vi "edit_coating(in).vi"(0 "Path":string) -> ()   [LabVIEW 2009]
uses:
  <vilib>/Utility/file.llb/Read From Spreadsheet File (string).vi
panel:
  in  "Recipe List":i32(listbox)
  out "error out":errorcluster
  out "Path Array":string[](array[string])
  out "Recipe":string[](array[string])
  in  "Coating Name :":string
  in  "Add Recipe":bool
  in  "ok":bool
  in  "cancel":bool
  in  "delete":bool
  in  "Move up":bool
  in  "Move down":bool
  in  "Coating":i32(listbox)
  out "OKTO":bool
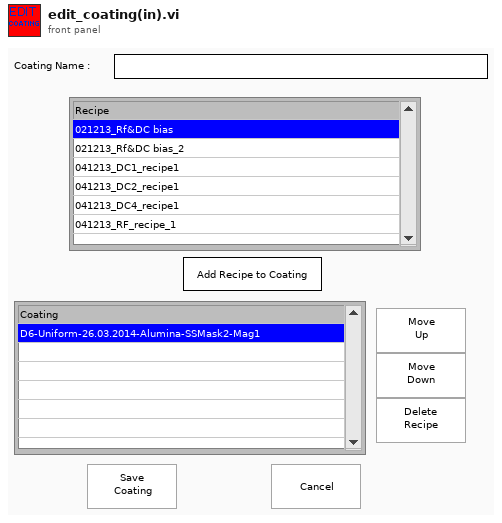
[diagram p1: front panel]
types:
  T1 = enum16{"open", "replace", "create", "open or create", "replace or create", "replace or create with confirmation"}
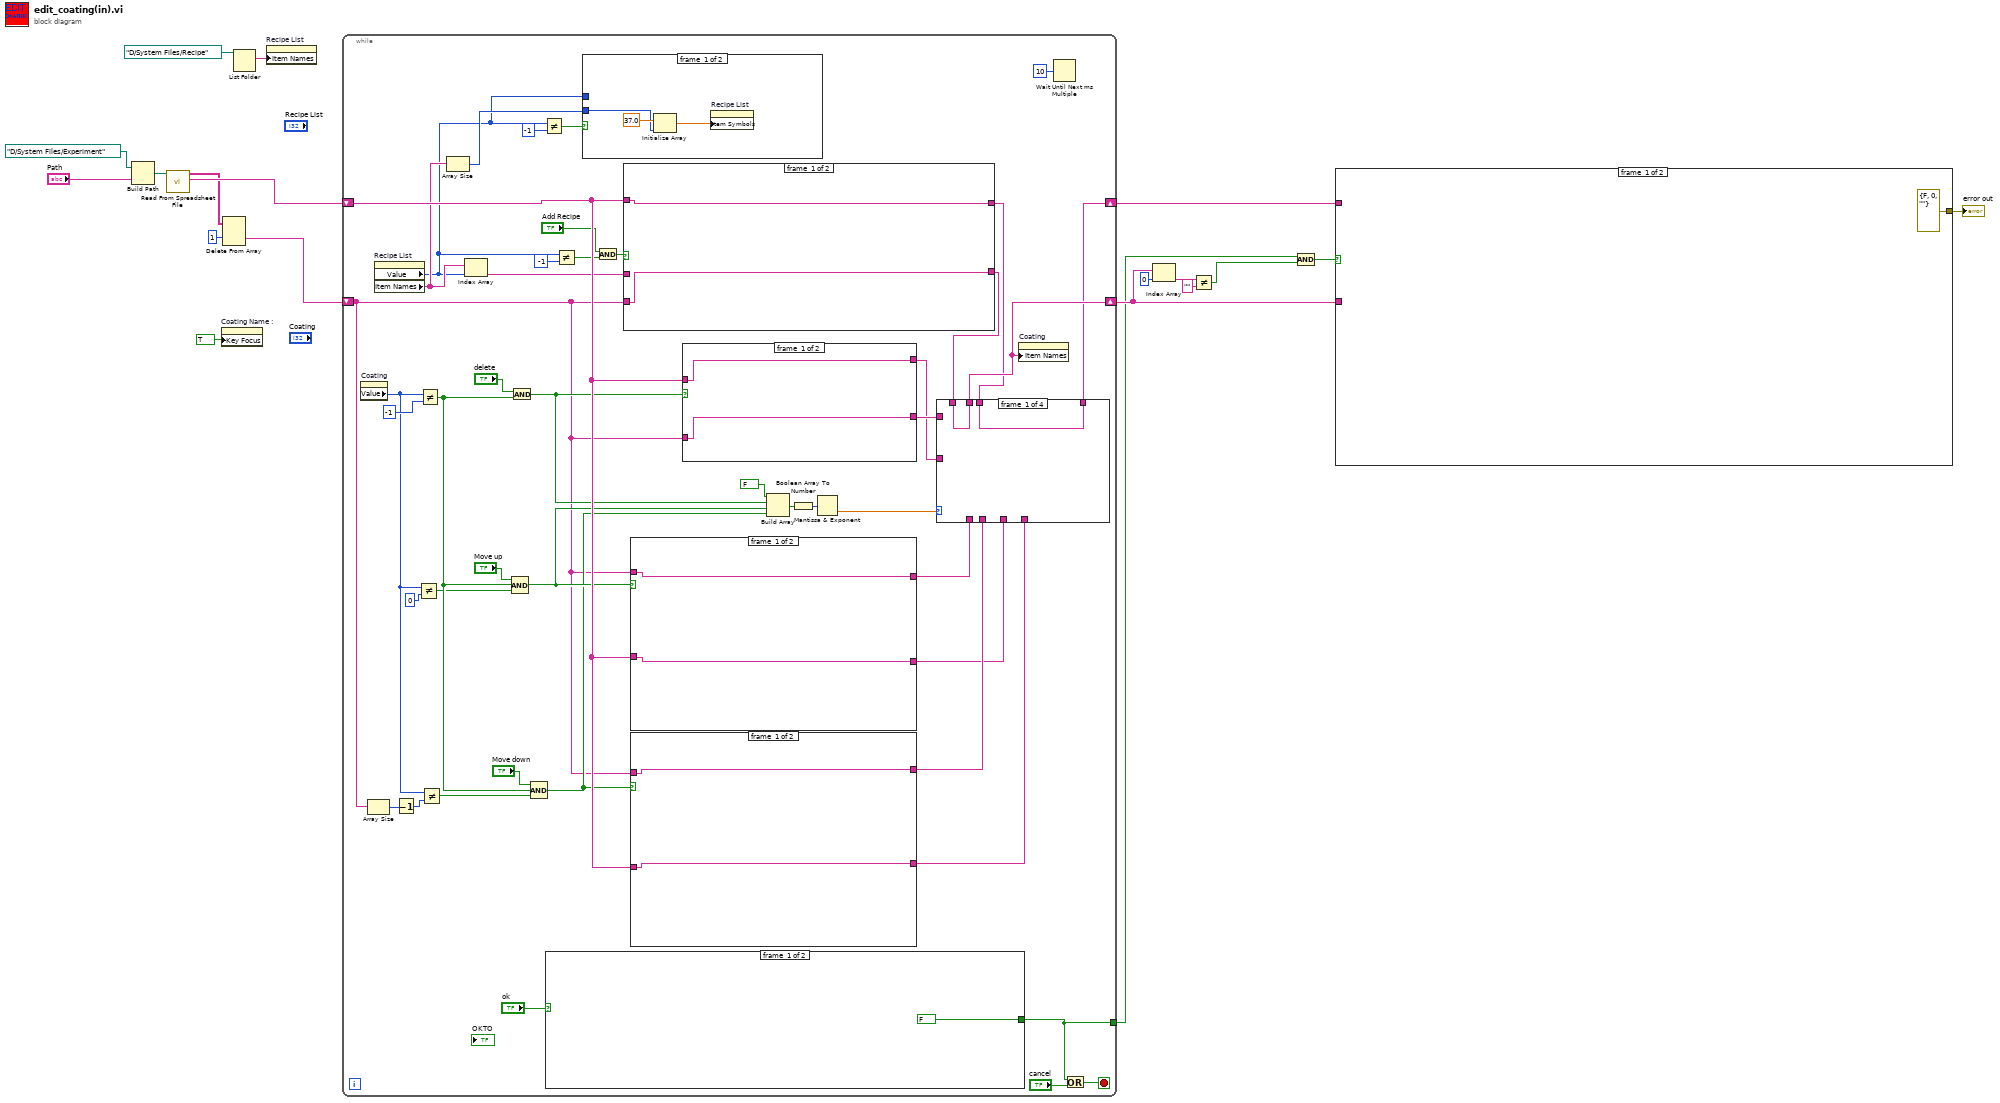
[diagram p0: block diagram]
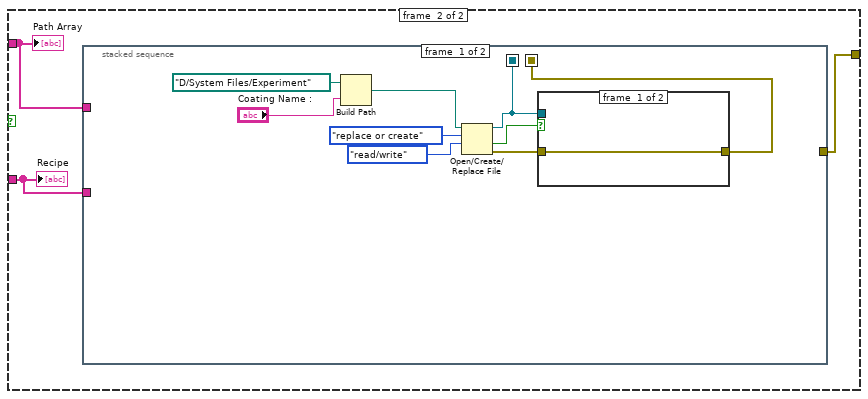
[diagram p2: hidden frame]
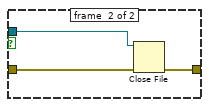
[diagram p3: hidden frame]
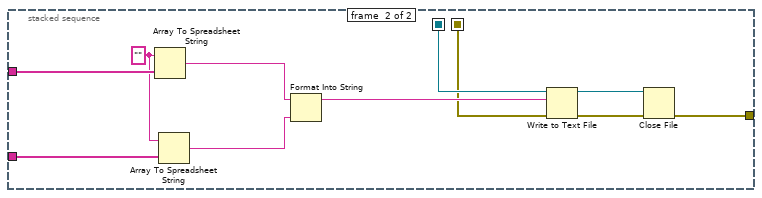
[diagram p4: hidden frame]
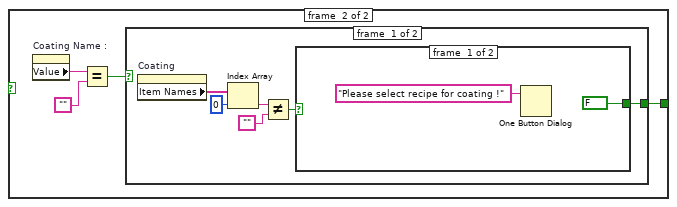
[diagram p5: hidden frame]
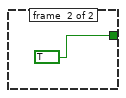
[diagram p6: hidden frame]
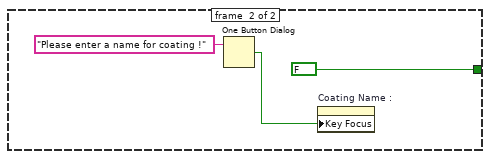
[diagram p7: hidden frame]
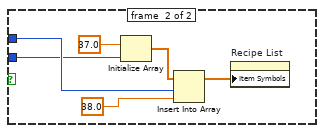
[diagram p8: hidden frame]
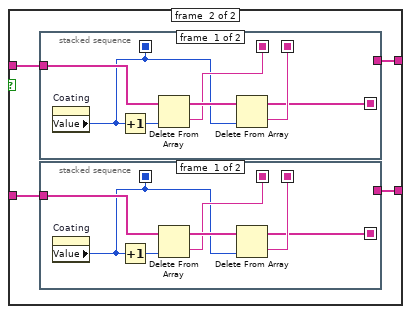
[diagram p12: hidden frame]
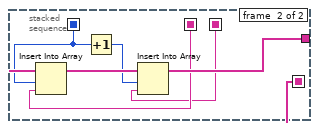
[diagram p13: hidden frame]
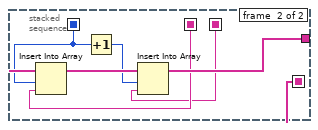
[diagram p14: hidden frame]
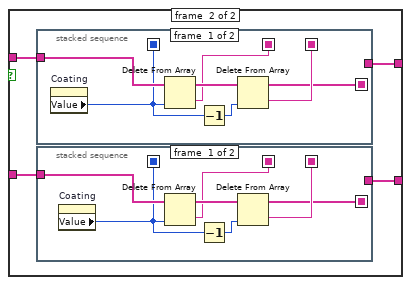
[diagram p15: hidden frame]
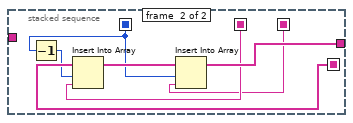
[diagram p16: hidden frame]
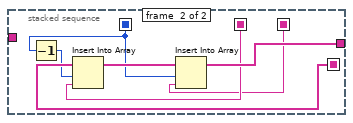
[diagram p17: hidden frame]
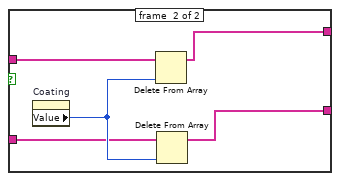
[diagram p18: hidden frame]
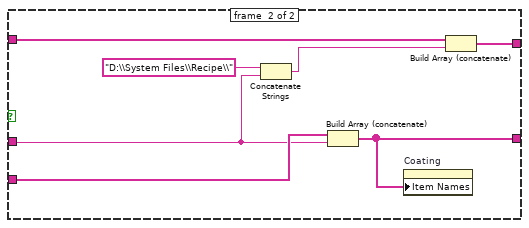
[diagram p19: hidden frame]
diagram:
  n1 = Build Path(base path=path "D:/System Files/Experiment", name or relative path="Path") -> (appended path=w19:path)
  n2 = call-poly <vilib>:"Read From Spreadsheet File.vi"("file path (dialog if empty)"=w19) -> ("first row"=w4:string[], "all rows"=w2:string[][])  [unwired: 6 in, 3 out]
  n3 = property on="Coating Name :" class="Str"("Key Focus"=TRUE) -> ()  [unwired: 2 in, 2 out]
  n4 = Delete From Array(array=w2, index (row)=1) -> (deleted portion=w1:string[])  [unwired: 2 in, 1 out]
  n5 = List Folder(path=path "D:/System Files/Recipe") -> (filenames=w8:string[])  [unwired: 3 in, 3 out]
  n6 = property on="Recipe List" class="LstBox (strict)"("Item Names"=w8) -> ()  [unwired: 2 in, 2 out]
  n7 = while {
    shift-right: [w51] -> w16
    shift-left: w4 -> [w54]
    shift-right: [w55] -> w15
    shift-left: w1 -> [w35]
    tunnel: [w21] -> w5
    stop <- w63 stop-if-true
    n8 = property on="Coating" class="LstBox (strict)"() -> ("Value"=w36:i32)  [unwired: 2 in, 2 out]
    n9 = Array Size(array=w35) -> (size(s)=w34:i32)
    n10 = property on="Recipe List" class="LstBox (strict)"() -> ("Value"=w23:i32, "Item Names"=w30:string[])  [unwired: 2 in, 2 out]
    n11 = Decrement(x=w34) -> (x-1=w33:i32)
    n12 = Not Equal?(x=w36, y=0) -> (x != y?=w38:bool)
    n13 = Not Equal?(x=w36, y=-1) -> (x != y?=w42:bool)
    n14 = Not Equal?(x=w36, y=w33) -> (x != y?=w37:bool)
    n15 = Array Size(array=w30) -> (size(s)=w28:i32)
    n16 = Index Array(array=w30, index=w23) -> (element=w32:string)
    n17 = And(x="delete", y=w42) -> (x .and. y?=w45:bool)
    n18 = Compound Arithmetic op=AND("Move up", w42, w38) -> (w43:bool)
    n19 = Compound Arithmetic op=AND("Move down", w42, w37) -> (w40:bool)
    n20 = Not Equal?(x=w23, y=-1) -> (x != y?=w29:bool)
    n21 = case shown="True" "ok" {
      tunnel: [FALSE w66] -> w21
      frame #0 {
      }
      frame #1 {
        n22 = property on="Coating Name :" class="Str"() -> ("Value"=w68:string)  [unwired: 2 in, 2 out]
        n23 = Equal?(x=w68, y="") -> (x = y?=w67:bool)
        n24 = case shown="True" w67 {
          tunnel: [w70 FALSE] -> w66
          frame #0 {
            n25 = property on="Coating" class="LstBox (strict)"() -> ("Item Names"=w73:string[])  [unwired: 2 in, 2 out]
            n26 = Index Array(array=w73, index=0) -> (element=w75:string)
            n27 = Not Equal?(x=w75, y="") -> (x != y?=w71:bool)
            n28 = case shown="False" w71 {
              tunnel: [FALSE TRUE] -> w70
              frame #0 {
                n29 = One Button Dialog(message="Please select recipe for coating !") -> ()  [unwired: 1 in, 1 out]
              }
              frame #1 {
              }
            }
          }
          frame #1 {
            n30 = One Button Dialog(message="Please enter a name for coating !") -> (true=w79:bool)  [unwired: 1 in]
            n31 = property on="Coating Name :" class="Str"("Key Focus"=w79) -> ()  [unwired: 2 in, 2 out]
          }
        }
      }
    }
    n32 = Not Equal?(x=w23, y=-1) -> (x != y?=w24:bool)
    n33 = case shown="False" w29 {
      tunnel: w23 -> [_ w87]
      tunnel: w28 -> [w83 w86]
      frame #0 {
        n34 = Initialize Array(37.0 ("element"), w83) -> (w82:dbl[])
        n35 = property on="Recipe List" class="LstBox (strict)"("Item Symbols"=w82) -> ()  [unwired: 2 in, 2 out]
      }
      frame #1 {
        n36 = Initialize Array(37.0 ("element"), w86) -> (w90:dbl[])
        n37 = Insert Into Array(array=w90, index=w87, new element=38.0 ("element")) -> (w85:dbl[])
        n38 = property on="Recipe List" class="LstBox (strict)"("Item Symbols"=w85) -> ()  [unwired: 2 in, 2 out]
      }
    }
    n39 = And(x="Add Recipe", y=w24) -> (x .and. y?=w26:bool)
    n40 = case shown="True" w26 {
      tunnel: [w175 w180] -> w52
      tunnel: [w174 w179] -> w53
      tunnel: w35 -> [w174 w182]
      tunnel: w54 -> [w175 w181]
      tunnel: w32 -> [_ w177]
      frame #0 {
      }
      frame #1 {
        n41 = Concatenate Strings("D:\\System Files\\Recipe\\" ("string"), w177) -> (w176:string)
        n42 = Build Array (concatenate)(w182, w177) -> (w179:string[])
        n43 = property on="Coating" class="LstBox (strict)"("Item Names"=w179) -> ()  [unwired: 2 in, 2 out]
        n44 = Build Array (concatenate)(w181, w176) -> (w180:string[])
      }
    }
    n45 = case shown="True" w43 {
      tunnel: w35 -> [w134 w138]
      tunnel: [w134 w137] -> w57
      tunnel: w54 -> [w133 w136]
      tunnel: [w133 w135] -> w50
      frame #0 {
      }
      frame #1 {
        n46 = stacked-sequence {
          seq-local: [w156 _] -> [_ w161]
          seq-local: [w155 _] -> [_ w160]
          seq-local: [w154 _] -> [_ w166]
          seq-local: [w153 _] -> [_ w163]
          tunnel: w138 -> [w159 _]
          tunnel: [_ w164] -> w137
          frame #0 {
            n47 = property on="Coating" class="LstBox (strict)"() -> ("Value"=w153:i32)  [unwired: 2 in, 2 out]
            n48 = Delete From Array(array=w159, index=w153) -> (deleted portion=w156:string, array with subset deleted=w158:string[])  [unwired: 1 in]
            n49 = Decrement(x=w153) -> (x-1=w157:i32)
            n50 = Delete From Array(array=w158, index=w157) -> (deleted portion=w155:string, array with subset deleted=w154:string[])  [unwired: 1 in]
          }
          frame #1 {
            n51 = Decrement(x=w163) -> (x-1=w162:i32)
            n52 = Insert Into Array(array=w166, index=w162, new element=w161) -> (w165:string[])
            n53 = Insert Into Array(array=w165, index=w163, new element=w160) -> (w164:string[])
          }
        }
        n54 = stacked-sequence {
          seq-local: [w142 _] -> [_ w147]
          seq-local: [w141 _] -> [_ w146]
          seq-local: [w140 _] -> [_ w152]
          seq-local: [w139 _] -> [_ w149]
          tunnel: w136 -> [w145 _]
          tunnel: [_ w150] -> w135
          frame #0 {
            n55 = property on="Coating" class="LstBox (strict)"() -> ("Value"=w139:i32)  [unwired: 2 in, 2 out]
            n56 = Delete From Array(array=w145, index=w139) -> (deleted portion=w142:string, array with subset deleted=w144:string[])  [unwired: 1 in]
            n57 = Decrement(x=w139) -> (x-1=w143:i32)
            n58 = Delete From Array(array=w144, index=w143) -> (deleted portion=w141:string, array with subset deleted=w140:string[])  [unwired: 1 in]
          }
          frame #1 {
            n59 = Decrement(x=w149) -> (x-1=w148:i32)
            n60 = Insert Into Array(array=w152, index=w148, new element=w147) -> (w151:string[])
            n61 = Insert Into Array(array=w151, index=w149, new element=w146) -> (w150:string[])
          }
        }
      }
    }
    n62 = case shown="True" w40 {
      tunnel: w35 -> [w100 w104]
      tunnel: [w100 w103] -> w56
      tunnel: w54 -> [w99 w102]
      tunnel: [w99 w101] -> w48
      frame #0 {
      }
      frame #1 {
        n63 = stacked-sequence {
          seq-local: [w121 _] -> [_ w129]
          seq-local: [w123 _] -> [_ w128]
          seq-local: [w122 _] -> [_ w132]
          seq-local: [w119 _] -> [_ w126]
          tunnel: w104 -> [w124 _]
          tunnel: [_ w131] -> w103
          frame #0 {
            n64 = property on="Coating" class="LstBox (strict)"() -> ("Value"=w119:i32)  [unwired: 2 in, 2 out]
            n65 = Increment(x=w119) -> (x+1=w120:i32)
            n66 = Delete From Array(array=w124, index=w120) -> (deleted portion=w121:string, array with subset deleted=w125:string[])  [unwired: 1 in]
            n67 = Delete From Array(array=w125, index=w119) -> (deleted portion=w123:string, array with subset deleted=w122:string[])  [unwired: 1 in]
          }
          frame #1 {
            n68 = Insert Into Array(array=w132, index=w126, new element=w129) -> (w130:string[])
            n69 = Increment(x=w126) -> (x+1=w127:i32)
            n70 = Insert Into Array(array=w130, index=w127, new element=w128) -> (w131:string[])
          }
        }
        n71 = stacked-sequence {
          seq-local: [w107 _] -> [_ w115]
          seq-local: [w109 _] -> [_ w114]
          seq-local: [w108 _] -> [_ w118]
          seq-local: [w105 _] -> [_ w112]
          tunnel: w102 -> [w110 _]
          tunnel: [_ w117] -> w101
          frame #0 {
            n72 = property on="Coating" class="LstBox (strict)"() -> ("Value"=w105:i32)  [unwired: 2 in, 2 out]
            n73 = Increment(x=w105) -> (x+1=w106:i32)
            n74 = Delete From Array(array=w110, index=w106) -> (deleted portion=w107:string, array with subset deleted=w111:string[])  [unwired: 1 in]
            n75 = Delete From Array(array=w111, index=w105) -> (deleted portion=w109:string, array with subset deleted=w108:string[])  [unwired: 1 in]
          }
          frame #1 {
            n76 = Insert Into Array(array=w118, index=w112, new element=w115) -> (w116:string[])
            n77 = Increment(x=w112) -> (x+1=w113:i32)
            n78 = Insert Into Array(array=w116, index=w113, new element=w114) -> (w117:string[])
          }
        }
      }
    }
    n79 = case shown="True" w45 {
      tunnel: w54 -> [w167 w173]
      tunnel: w35 -> [w168 w171]
      tunnel: [w168 w170] -> w58
      tunnel: [w167 w169] -> w49
      frame #0 {
      }
      frame #1 {
        n80 = property on="Coating" class="LstBox (strict)"() -> ("Value"=w172:i32)  [unwired: 2 in, 2 out]
        n81 = Delete From Array(array=w173, index=w172) -> (array with subset deleted=w169:string[])  [unwired: 1 in, 1 out]
        n82 = Delete From Array(array=w171, index=w172) -> (array with subset deleted=w170:string[])  [unwired: 1 in, 1 out]
      }
    }
    n83 = Build Array(FALSE, w45, w43, w40) -> (w60:bool[])
    n84 = Boolean Array To Number(Boolean array=w60) -> (number=w61:u32)
    n85 = Mantissa & Exponent(0:w61) -> (2:w59:dbl)  [unwired: 1 out]
    n86 = case shown="0, Default" w59 {
      tunnel: w58 -> [_ w94 _ _]
      tunnel: [w92 w94 w96 w98] -> w55
      tunnel: w57 -> [_ _ w96 _]
      tunnel: w56 -> [_ _ _ w98]
      tunnel: w53 -> [w92 _ _ _]
      tunnel: w52 -> [w91 _ _ _]
      tunnel: [w91 w93 w95 w97] -> w51
      tunnel: w50 -> [_ _ w95 _]
      tunnel: w49 -> [_ w93 _ _]
      tunnel: w48 -> [_ _ _ w97]
      frame #0 {
      }
      frame #1 {
      }
      frame #2 {
      }
      frame #3 {
      }
    }
    n87 = property on="Coating" class="LstBox (strict)"("Item Names"=w55) -> ()  [unwired: 2 in, 2 out]
    n88 = Wait Until Next ms Multiple(millisecond multiple=u32 10) -> ()  [unwired: 1 out]
    n89 = Or(x=w21, y="cancel") -> (x .or. y?=w63:bool)
  }
  n90 = Index Array(array=w15, index=0) -> (element=w13:string)
  n91 = Not Equal?(x=w13, y="") -> (x != y?=w11:bool)
  n92 = Compound Arithmetic op=AND(w5, w11) -> (w10:bool)
  n93 = case shown="True" w10 {
    tunnel: w16 -> [_ w185]
    tunnel: w15 -> [_ w186]
    tunnel: [errorcluster {"status"=FALSE, "code"=0, "source"=""} ("error out") w184] -> w9
    frame #0 {
    }
    frame #1 {
      n94 = stacked-sequence {
        seq-local: [w192 _] -> [_ w205]
        seq-local: [w190 _] -> [_ w201]
        tunnel: w185 -> [_ w210]
        tunnel: w186 -> [_ w209]
        tunnel: [_ w200] -> w184
        frame #0 {
          n95 = Build Path(base path=path "D:/System Files/Experiment" ("start path"), name or relative path="Coating Name :") -> (appended path=w187:path)
          n96 = Open/Create/Replace File(file path (use dialog)=w187, operation (0:open)=T1."replace or create", access (0:read/write)=enum16{"read/write", "read-only", "write-only"}."read/write") -> (refnum out=w192:refnum<file>, cancelled=w194:bool, error out=w191:errorcluster)  [unwired: 3 in]
          n97 = case shown="True" w194 {
            tunnel: w192 -> [_ w199]
            tunnel: w191 -> [w196 w198]
            tunnel: [w196 w197] -> w190
            frame #0 {
            }
            frame #1 {
              n98 = Close File(refnum=w199, error in=w198) -> (error out=w197:errorcluster)  [unwired: 1 out]
            }
          }
        }
        frame #1 {
          w204 = "" ("format string")
          n99 = Array To Spreadsheet String(array=w210, 3:w204) -> (spreadsheet string=w208:string)  [unwired: 1 in]
          n100 = Array To Spreadsheet String(array=w209, 3:w204) -> (spreadsheet string=w207:string)  [unwired: 1 in]
          n101 = Format Into String(initial string=w208, w207) -> (resulting string=w206:string)  [unwired: 2 in, 1 out]
          n102 = Write to Text File(file (use dialog)=w205, text=w206, error in=w201) -> (refnum out=w202:refnum<file>, error out=w203:errorcluster)  [unwired: 1 in, 1 out]
          n103 = Close File(refnum=w202, error in=w203) -> (error out=w200:errorcluster)  [unwired: 1 out]
        }
      }
      "Path Array" <- w185
      "Recipe" <- w186
    }
  }
  "error out" <- w9
